vi "holoPathEditor.vi"(7 "Display":i32=1, 8 "error in":errorcluster, 9 "prev. Path":path, 10 "input cluster":T1={"1_Radio"=enum."Radio Selection 3", "1_Trans"=0.0, "1_Phase"=0.0, "1_HoloCode"="", "1_Semi"=FALSE, "1_Active"=0, "1_ModType"="", "1_Flip"="", "HoloNum"=0.0, "paramStr"="", "paramVal"=0, "paramAux"=""}) -> (0 "error out":errorcluster, 1 "active?":bool, 2 "file or folder exists?":bool, 3 "appended path":path)   [LabVIEW 2023]
panel:
  # "Display=0 means \"beam explorator\""
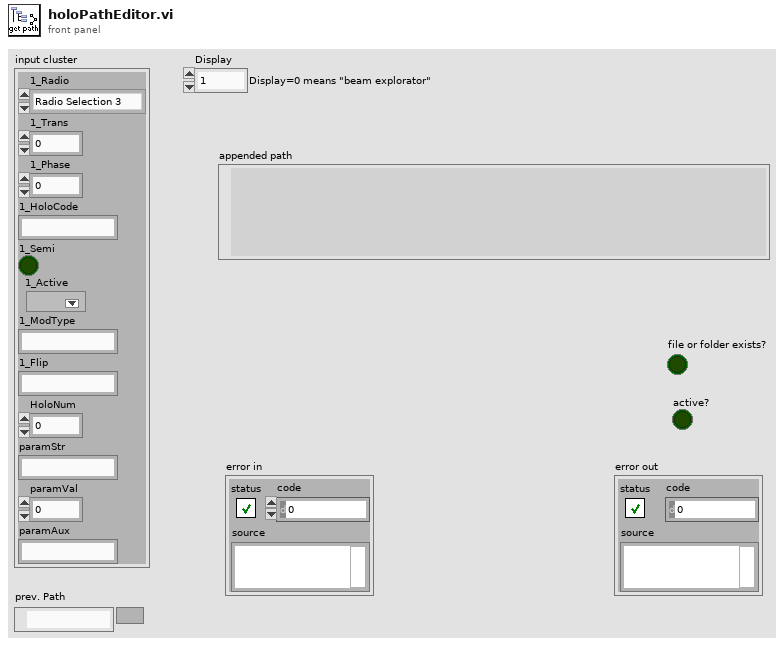
[diagram p1: front panel]
types:
  T1 = cluster{"1_Radio":enum32{"Radio Selection 1", "Radio Selection 2", "Radio Selection 3", "Radio Selection 4", "Radio Selection 5", "Radio Selection 6", "Radio Selection 7", "Radio Selection 8"}, "1_Trans":dbl, "1_Phase":dbl, "1_HoloCode":string, "1_Semi":bool, "1_Active":u16, "1_ModType":string, "1_Flip":string, "HoloNum":dbl, "paramStr":string, "paramVal":i64, "paramAux":string}
  T2 = enum32{"Radio Selection 1", "Radio Selection 2", "Radio Selection 3", "Radio Selection 4", "Radio Selection 5", "Radio Selection 6", "Radio Selection 7", "Radio Selection 8"}
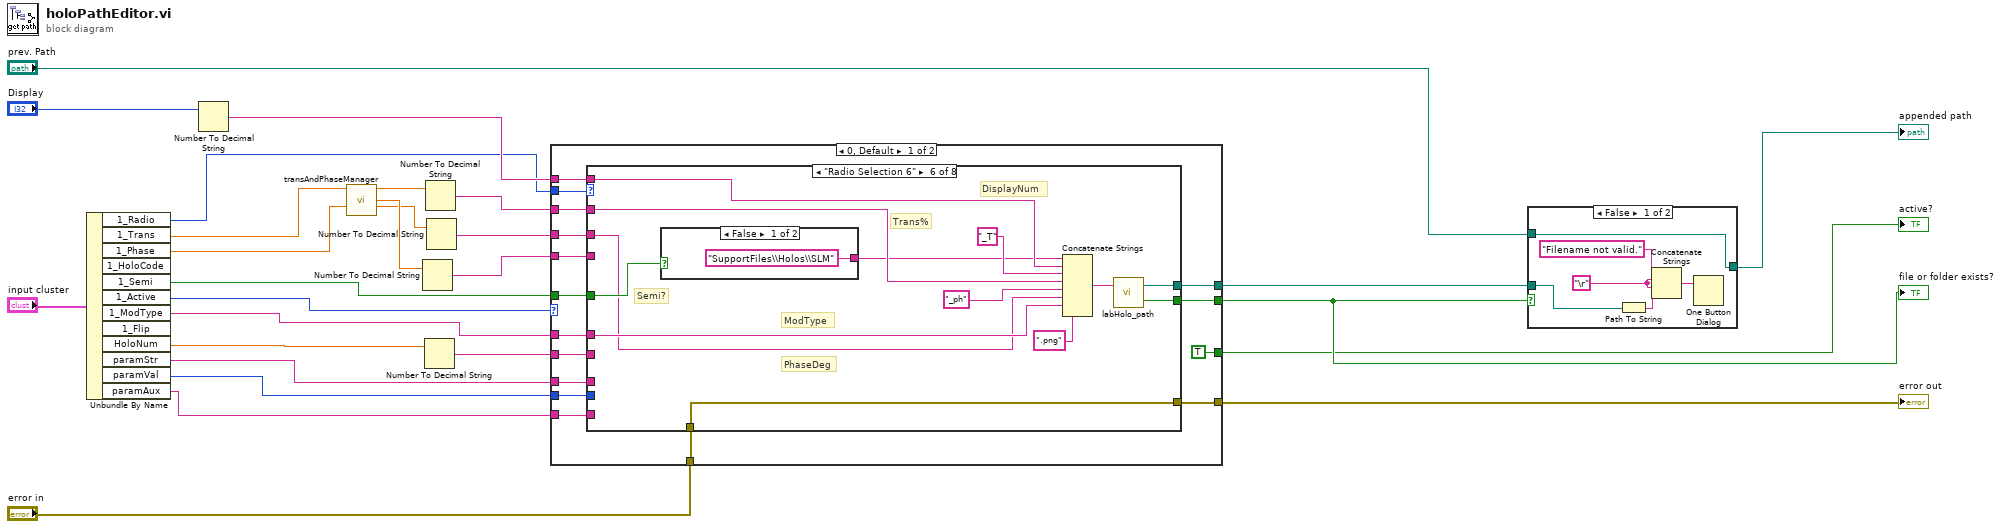
[diagram p0: block diagram]
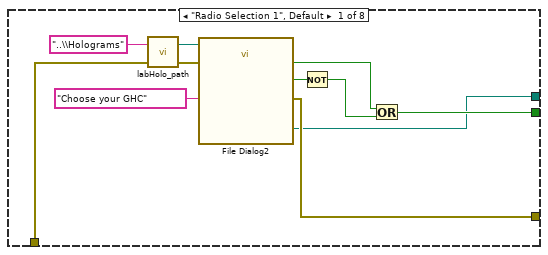
[diagram p3: hidden frame]
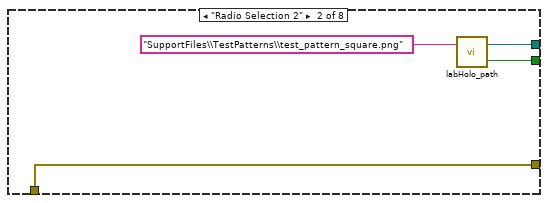
[diagram p4: hidden frame]
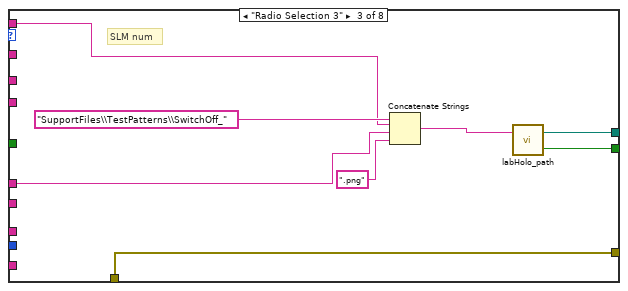
[diagram p5: hidden frame]
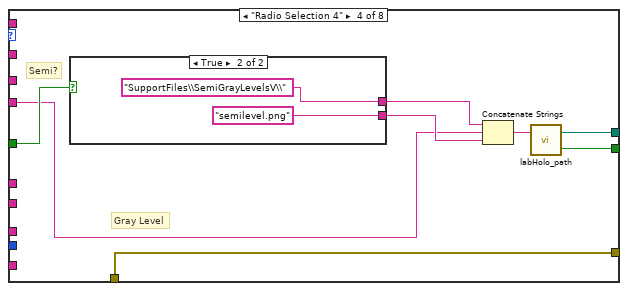
[diagram p6: hidden frame]
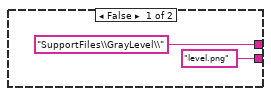
[diagram p7: hidden frame]
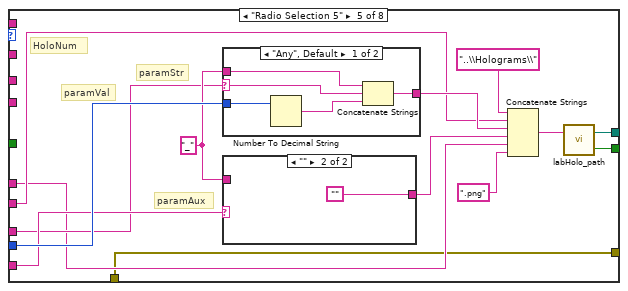
[diagram p8: hidden frame]
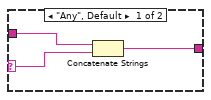
[diagram p9: hidden frame]
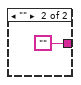
[diagram p10: hidden frame]
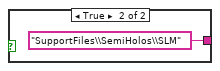
[diagram p11: hidden frame]
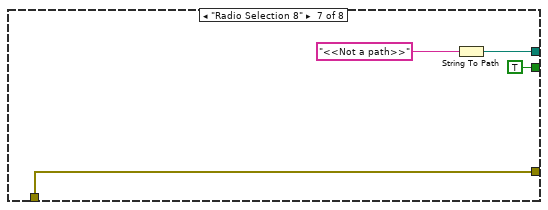
[diagram p12: hidden frame]
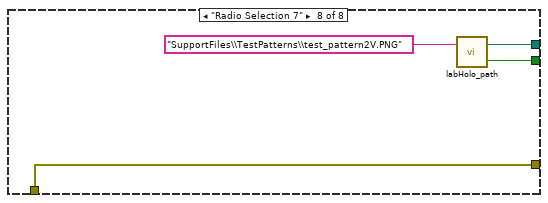
[diagram p13: hidden frame]
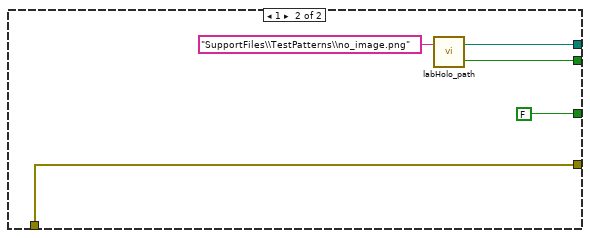
[diagram p14: hidden frame]
diagram:
  n1 = Unbundle By Name("input cluster") -> ("1_Radio"=w13:T2, "1_Trans"=w21:dbl, "1_Phase"=w20:dbl, "1_Semi"=w12:bool, "1_Active"=w11:u16, "1_ModType"=w10:string, "HoloNum"=w24:dbl, "paramStr"=w8:string, "paramVal"=w22:i64, "paramAux"=w9:string)  [unwired: 2 out]
  n2 = Number To Decimal String(number="Display") -> (decimal integer string=w25:string)  [unwired: 1 in]
  n3 = call "transAndPhaseManager.vi"("Trans in"=w21, "Phase in"=w20) -> ("Trans %"=w15:dbl, "T gl"=w19:dbl, "Phase Deg"=w17:dbl)  [unwired: 9 in, 2 out]
  n4 = Number To Decimal String(number=w19) -> (decimal integer string=w18:string)  [unwired: 1 in]
  n5 = Number To Decimal String(number=w24) -> (decimal integer string=w23:string)  [unwired: 1 in]
  n6 = Number To Decimal String(number=w15) -> (decimal integer string=w14:string)  [unwired: 1 in]
  n7 = Number To Decimal String(number=w17) -> (decimal integer string=w16:string)  [unwired: 1 in]
  n8 = case shown="0, Default" w11 {
    tunnel: w13 -> [w43 _]
    tunnel: [w42 w128] -> w4
    tunnel: w25 -> [w41 _]
    tunnel: w12 -> [w40 _]
    tunnel: w23 -> [w39 _]
    tunnel: w8 -> [w38 _]
    tunnel: w9 -> [w37 _]
    tunnel: w22 -> [w36 _]
    tunnel: w10 -> [w35 _]
    tunnel: w18 -> [w34 _]
    tunnel: w16 -> [w33 _]
    tunnel: w14 -> [w32 _]
    tunnel: "error in" -> [w31 w127]
    tunnel: [w30 w127] -> w5
    tunnel: [w29 w126] -> w3
    tunnel: [TRUE FALSE] -> w1
    frame 0, Default {
      n9 = case shown="\"Radio Selection 6\"" w43 {
        tunnel: [w46 w56 w64 w70 w86 w113 w120 w123] -> w42
        tunnel: w41 -> [_ _ w59 _ _ w107 _ _]
        tunnel: w40 -> [_ _ _ w69 _ w110 _ _]
        tunnel: w39 -> [_ _ _ _ w82 _ _ _]
        tunnel: w38 -> [_ _ _ _ w81 _ _ _]
        tunnel: w37 -> [_ _ _ _ w83 _ _ _]
        tunnel: w36 -> [_ _ _ _ w87 _ _ _]
        tunnel: w35 -> [_ _ w58 _ w80 w105 _ _]
        tunnel: w34 -> [_ _ _ w68 _ _ _ _]
        tunnel: w33 -> [_ _ _ _ _ w104 _ _]
        tunnel: w32 -> [_ _ _ _ _ w109 _ _]
        tunnel: w31 -> [w50 w55 w62 w67 w79 w103 w118 w122]
        tunnel: [w49 w55 w62 w67 w79 w103 w118 w122] -> w30
        tunnel: [w47 w54 w61 w66 w78 w102 TRUE ("Exists?") w121] -> w29
        frame "Radio Selection 1", Default {
          n10 = call "labHolo_path.vi"("sub folder or file (str)"="..\\Holograms" ("name or relative path")) -> ("labHolo path"=w51:path)  [unwired: 1 in, 1 out]
          n11 = call "File Dialog2"("start path"=w51, "prompt"="Choose your GHC", "error in"=w50) -> ("selected path"=w46:path, "exists"=w48:bool, "cancelled"=w45:bool, "error out"=w49:errorcluster)  [unwired: 9 in]
          n12 = Not(x=w45) -> (.not. x?=w44:bool)
          n13 = Or(x=w48, y=w44) -> (x .or. y?=w47:bool)
        }
        frame "Radio Selection 2" {
          n14 = call "labHolo_path.vi"("sub folder or file (str)"="SupportFiles\\TestPatterns\\test_pattern_square.png" ("name or relative path")) -> ("Exists?"=w54:bool, "labHolo path"=w56:path)  [unwired: 1 in]
        }
        frame "Radio Selection 3" {
          # "SLM num"
          n15 = Concatenate Strings("SupportFiles\\TestPatterns\\SwitchOff_" ("name or relative path"), w59, w58, ".png" ("string")) -> (w63:string)
          n16 = call "labHolo_path.vi"("sub folder or file (str)"=w63) -> ("Exists?"=w61:bool, "labHolo path"=w64:path)  [unwired: 1 in]
        }
        frame "Radio Selection 4" {
          # "Semi?"
          # "Gray Level"
          n17 = case shown="True" w69 {
            tunnel: ["SupportFiles\\GrayLevel\\" ("name or relative path") "SupportFiles\\SemiGrayLevelsV\\" ("name or relative path")] -> w73
            tunnel: ["level.png" ("name or relative path") "semilevel.png" ("name or relative path")] -> w72
            frame False {
            }
            frame True {
            }
          }
          n18 = Concatenate Strings(w73, w68, w72) -> (w71:string)
          n19 = call "labHolo_path.vi"("sub folder or file (str)"=w71) -> ("Exists?"=w66:bool, "labHolo path"=w70:path)  [unwired: 1 in]
        }
        frame "Radio Selection 5" {
          w84 = "_" ("string")
          # "HoloNum"
          # "paramAux"
          # "paramVal"
          # "paramStr"
          n20 = case shown="\"Any\", Default" w81 {
            selector: w81 -> [w98 _]
            tunnel: [w99 ""] -> w89
            tunnel: w84 -> [w97 _]
            tunnel: w87 -> [w96 _]
            frame "Any", Default {
              n21 = Number To Decimal String(number=w96) -> (decimal integer string=w100:string)  [unwired: 1 in]
              n22 = Concatenate Strings(w97, w98, w100) -> (w99:string)
            }
            frame "" {
            }
          }
          n23 = case shown="\"\"" w83 {
            selector: w83 -> [w93 _]
            tunnel: [w94 ""] -> w88
            tunnel: w84 -> [w92 _]
            frame "Any", Default {
              n24 = Concatenate Strings(w92, w93) -> (w94:string)
            }
            frame "" {
            }
          }
          n25 = Concatenate Strings("..\\Holograms\\" ("string"), w82, w89, w88, w80, ".png" ("string")) -> (w91:string)
          n26 = call "labHolo_path.vi"("sub folder or file (str)"=w91) -> ("Exists?"=w78:bool, "labHolo path"=w86:path)  [unwired: 1 in]
        }
        frame "Radio Selection 6" {
          # "Semi?"
          # "PhaseDeg"
          # "ModType"
          # "Trans%"
          # "DisplayNum"
          n27 = case shown="False" w110 {
            tunnel: ["SupportFiles\\Holos\\SLM" ("name or relative path") "SupportFiles\\SemiHolos\\SLM" ("name or relative path")] -> w106
            frame False {
            }
            frame True {
            }
          }
          n28 = Concatenate Strings(w106, w107, "_T" ("string"), w109, "_ph" ("string"), w104, w105, ".png" ("Master Thesis (folder)")) -> (w114:string)
          n29 = call "labHolo_path.vi"("sub folder or file (str)"=w114) -> ("Exists?"=w102:bool, "labHolo path"=w113:path)  [unwired: 1 in]
        }
        frame "Radio Selection 8" {
          n30 = String To Path(string="<<Not a path>>" ("name or relative path")) -> (path=w120:path)
        }
        frame "Radio Selection 7" {
          n31 = call "labHolo_path.vi"("sub folder or file (str)"="SupportFiles\\TestPatterns\\test_pattern2V.PNG" ("name or relative path")) -> ("Exists?"=w121:bool, "labHolo path"=w123:path)  [unwired: 1 in]
        }
      }
    }
    frame 1 {
      n32 = call "labHolo_path.vi"("sub folder or file (str)"="SupportFiles\\TestPatterns\\no_image.png" ("name or relative path")) -> ("Exists?"=w126:bool, "labHolo path"=w128:path)  [unwired: 1 in]
    }
  }
  "file or folder exists?" <- w3
  "error out" <- w5
  "active?" <- w1
  n33 = case shown="False" w3 {
    tunnel: [w135 w136] -> w7
    tunnel: w4 -> [w133 w136]
    tunnel: "prev. Path" -> [w135 _]
    frame False {
      w131 = "\r"
      n34 = Path To String(path=w133) -> (string=w132:string)
      n35 = Concatenate Strings("Filename not valid." ("message"), w131, w131, w132) -> (w134:string)
      n36 = One Button Dialog(message=w134) -> ()  [unwired: 1 in, 1 out]
    }
    frame True {
    }
  }
  "appended path" <- w7
